vi "OE2011&OE2021_Data Index.vi"(1 "Parameter Type":u16(ring) items=["Xh1", "Yh1", "Xh1_Noise", "Yh1_Noise", "Rh1", "θh1", "Xh2", "Yh2", "Rh2", "θh2", "Xh3", "Yh3", "Rh3", "θh3", "Xh4", "Yh4", "Rh4", "θh4", "Xh5", "Yh5", "Rh5", "θh5", "Xh5_Noise", "Yh5_Noise", "Xh6", "Yh6", "Rh6", "θh6", "Xh7", "Yh7", "Rh7", "θh7", "Xh8", "Yh8", "Rh8", "θh8", "OSC1_Frequency", "OSC2_Frequency", "AUX-IN1", "AUX-IN2", "AUX-IN3", "AUX-IN4"], 2 "Input Date Array":dbl[](array[numeric])) -> (0 "Parameter":dbl)   [LabVIEW 2011]
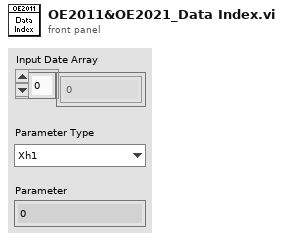
[diagram p1: front panel]
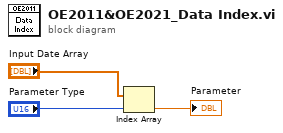
[diagram p0: block diagram]
diagram:
  n1 = Index Array(array="Input Date Array", index="Parameter Type") -> (element=→"Parameter":dbl)
